vi "Get CAN Configuration.vi"(8 "error in (no error)":errorcluster, 11 "Ethernet in":refnum<class "ENET_BS1201.lvclass">) -> (0 "error out":errorcluster, 1 "Configuration Error?":bool, 2 "CAN Settings":T1, 3 "Ethernet out":refnum<class "ENET_BS1201.lvclass">)   [LabVIEW 2021, in "BS120x Driver.lvlib" / "ENET_BS1201.lvclass"]
doc: "Retrieve Battery Simulator 1200 CAN settings.\n(c) 2019 Bloomy Controls, Inc. All rights reserved."
uses:
  ENET_BS1201.lvclass
  TypeDefs/CAN Settings.ctl
  ENET_BS1201.lvclass/ENET_BS1201.ctl
  BS120x.lvclass
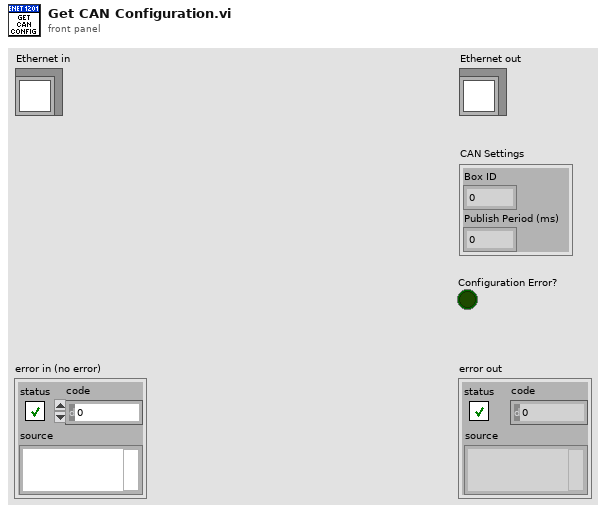
[diagram p1: front panel]
types:
  T1 = typedef "BS120x Driver.lvlib/BS120x.lvclass/CAN Settings.ctl" = cluster{"Box ID":i32, "Publish Period (ms)":i32}
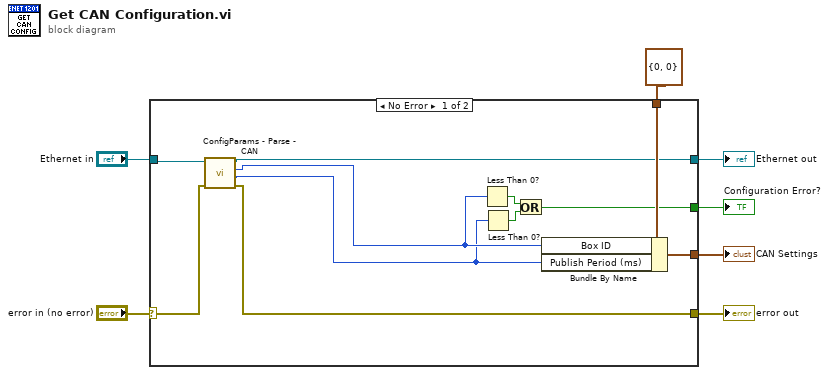
[diagram p0: block diagram]
diagram:
  n1 = case shown="No Error" "error in (no error)" {
    selector: "error in (no error)" -> [w11 w21]
    tunnel: [w10 w21] -> w6
    tunnel: [w13 w20] -> w4
    tunnel: "Ethernet in" -> [w12 w20]
    tunnel: [w17 w19] -> w2
    tunnel: T1 {"Box ID"=0, "Publish Period (ms)"=0} ("CAN Settings") -> [w18 w19]
    tunnel: [w14 _] -> w1
    frame No Error {
      n2 = call-dynamic "ConfigParams - Parse - CAN.vi"("error in (no error)"=w11, "Ethernet in"=w12) -> ("error out"=w10:errorcluster, "WritePeriod_ms"=w8:i32, "BoxID"=w9:i32, "Ethernet out"=w13:refnum<class "ENET_BS1201.lvclass">)  [unwired: 6 in]
      n3 = Less Than 0?(x=w9) -> (x < 0?=w16:bool)
      n4 = Less Than 0?(x=w8) -> (x < 0?=w15:bool)
      n5 = Or(x=w16, y=w15) -> (x .or. y?=w14:bool)
      n6 = Bundle By Name(cluster=w18, "Box ID"=w9, "Publish Period (ms)"=w8) -> (w17:T1)
    }
    frame Error {
    }
  }
  "error out" <- w6
  "Ethernet out" <- w4
  "CAN Settings" <- w2
  "Configuration Error?" <- w1
